vi "Student t Inverse CDF.vi"(10 "k degrees of freedom":i32=1, 11 "cdf(x)":dbl) -> (0 "error":i32, 3 "x":dbl)   [LabVIEW 2020, in "NI_Gmath.lvlib"]
doc: "Computes the continuous inverse cumulative distribution function (CDF) of the various distributions. You must manually select the polymorphic instance to use."
uses:
  NI_Gmath.lvlib
  st_error_code.ctl
panel:
  # "Student t Inverse CDF"
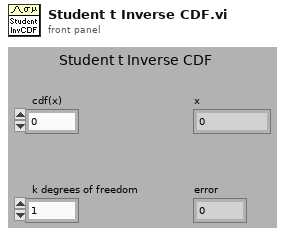
[diagram p1: front panel]
types:
  T1 = typedef "NI_Gmath.lvlib/st_error_code.ctl" = i32
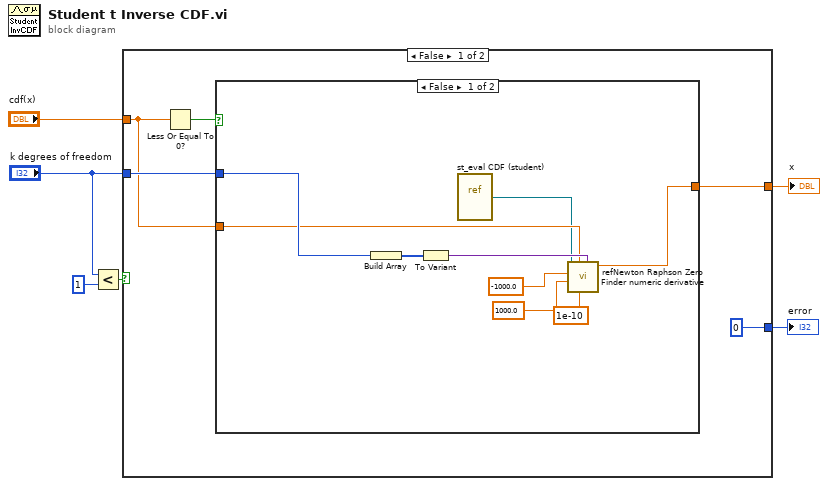
[diagram p0: block diagram]
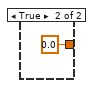
[diagram p2: hidden frame]
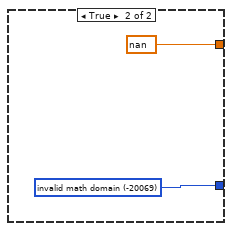
[diagram p3: hidden frame]
diagram:
  n1 = Less?(x="k degrees of freedom", y=1) -> (x < y?=w3:bool)
  n2 = case shown="False" w3 {
    tunnel: [0 ("invalid math domain") w22] -> w6
    tunnel: [w10 nan] -> w5
    tunnel: "cdf(x)" -> [w8 _]
    tunnel: "k degrees of freedom" -> [w9 _]
    frame False {
      n3 = Less Or Equal To 0?(x=w8) -> (x <= 0?=w7:bool)
      n4 = case shown="False" w7 {
        tunnel: [w17 0.0] -> w10
        tunnel: w8 -> [w16 _]
        tunnel: w9 -> [w18 _]
        frame False {
          n5 = Build Array(w18) -> (w20:i32[])
          n6 = To Variant(anything=w20) -> (Variant=w19:variant)
          n7 = vi-ref "st_eval CDF (student).vi"() -> ("vi reference"=w12:refnum<vi>)
          n8 = call "refNewton Raphson Zero Finder numeric derivative.vi"("function parameters"=w19, "accuracy"=1e-10, "level"=w16, "end"=1000.0 ("start"), "start"=-1000.0, "function refnum"=w12) -> ("zero"=w17:dbl)  [unwired: 2 in, 3 out]
        }
        frame True {
        }
      }
    }
    frame True {
      w22 = T1 -20069 items=["invalid math domain"=-20069, "Fourier interpolation size m >= n"=-20070, "empty array"=-20003] ("stat interp error code")
    }
  }
  "x" <- w5
  "error" <- w6
